vi "Delay.vi"(8 "error in (no error)":errorcluster, 9 "Data Flow Input":i32, 10 "Boolean In":bool, 11 "milliseconds to wait (10)":u32=10) -> (0 "error out":errorcluster, 2 "Boolean Out":bool)   [LabVIEW 2015]
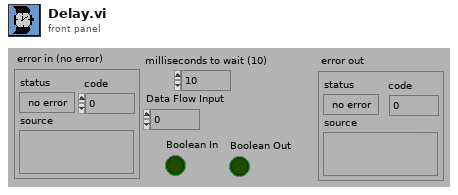
[diagram p1: front panel]
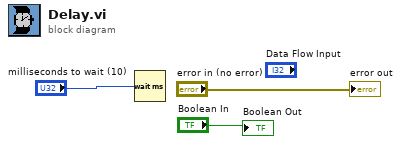
[diagram p0: block diagram]
diagram:
  n1 = Wait (ms)(milliseconds to wait="milliseconds to wait (10)") -> ()  [unwired: 1 out]
  "error out" <- "error in (no error)"
  "Boolean Out" <- "Boolean In"
